vi "DuraFET_pH_CalibCalc.vi"(1 "Eint: (mean voltage)":dbl=0.1318204577803552, 2 "Directemp (C)":dbl, 3 "Eext (REF or Vg)":dbl=1.0) -> (0 "pHint_tot":dbl=9.677584089217062)   [LabVIEW 2018]
panel:
  out "pHext_tot":dbl=nan
  in  "Salinity":dbl
  out "E0ext25":dbl=-inf format="%#_3g"
  out "E0int25":dbl=-0.4202114127602252 format="%#_3g"
  in  "calsal":dbl
  in  "calT":dbl=22.327
  in  "calpH":dbl=9.3
  in  "calEint":dbl=0.127974
  in  "calEext (const)":dbl=1.0
  # "pH Calibration (returns calib. coeff's)"
  # "pH Calculation (returns pHint & pHext)"
  # "INPUTS"
  # "INPUTS"
  # "OUTPUTS"
  # "OUTPUTS"
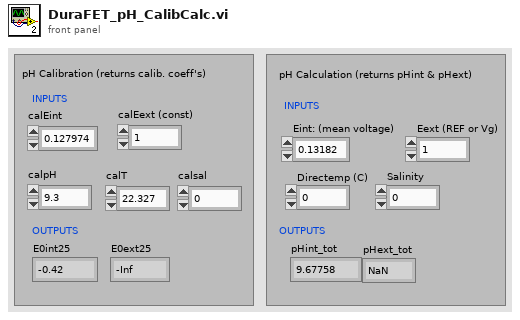
[diagram p1: front panel]
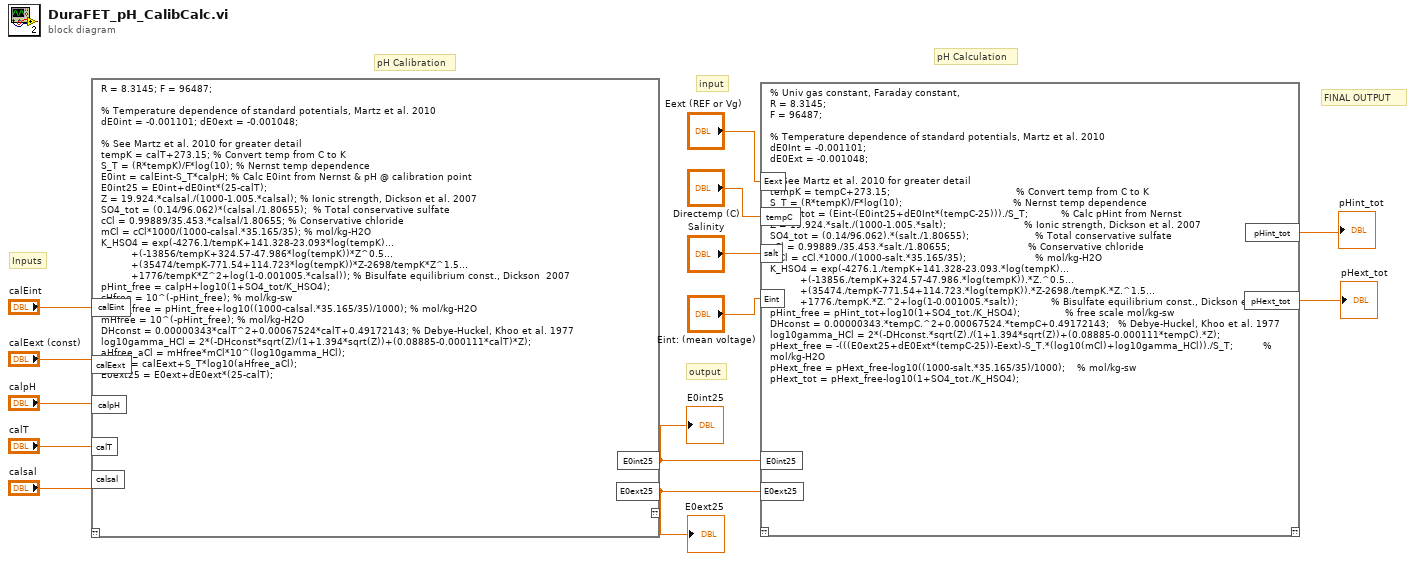
[diagram p0: block diagram]
diagram:
  # "Inputs"
  # "output"
  # "FINAL OUTPUT"
  # "input"
  # "pH Calculation"
  # "pH Calibration"
  n1 = script code="R = 8.3145; F = 96487; \n\n% Temperature dependence of standard potentials, Martz et al. 2010\ndE0int = -0.001101; dE0ext = -0.001048;\n\n% See Martz et al. 2010 for greater detail\ntempK = calT+273.15; % Convert temp from C to K\nS_T = (R*tempK)/F*log(10); % Nernst temp dependence\nE0int = calEint-S_T*calpH; % Calc E0int from Nernst & pH @ calibration point\nE0int25 = E0int+dE0int*(25-calT);\nZ = 19.924.*calsal./(1000-1.005.*calsal); % Ionic strength, Dickson et al. 2007\nSO4_tot = (0.14/96.062)*(calsal./1.80655);  % Total conservative sulfate\ncCl = 0.99889/35.453.*calsal/1.80655; % Conservative chloride\nmCl = cCl*1000/(1000-calsal.*35.165/35); % mol/kg-H2O\nK_HSO4 = exp(-4276.1/tempK+141.328-23.093*log(tempK)...\n          +(-13856/tempK+324.57-47.986*log(tempK))*Z^0.5...\n          +(35474/tempK-771.54+114.723*log(tempK))*Z-2698/tempK*Z^1.5...\n          +1776/tempK*Z^2+log(1-0.001005.*calsal)); % Bisulfate equilibrium const., Dickson  2007\npHint_free = calpH+log10(1+SO4_tot/K_HSO4);\ncHfree = 10^(-pHint_free); % mol/kg-sw\npHint_free = pHint_free+log10((1000-calsal.*35.165/35)/1000); % mol/kg-H2O\nmHfree = 10^(-pHint_free); % mol/kg-H2O\nDHconst = 0.00000343*calT^2+0.00067524*calT+0.49172143; % Debye-Huckel, Khoo et al. 1977\nlog10gamma_HCl = 2*(-DHconst*sqrt(Z)/(1+1.394*sqrt(Z))+(0.08885-0.000111*calT)*Z);\naHfree_aCl = mHfree*mCl*10^(log10gamma_HCl); \nE0ext = calEext+S_T*log10(aHfree_aCl);\nE0ext25 = E0ext+dE0ext*(25-calT);"("calEint"="calEint", "calEext"="calEext (const)", "calpH"="calpH", "calT"="calT", "calsal"="calsal") -> ("E0int25"=w3:cdb, "E0ext25"=w4:cdb)  [unwired: 1 in, 1 out]
  "E0int25" <- w3
  "E0ext25" <- w4
  n2 = script code="% Univ gas constant, Faraday constant, \nR = 8.3145;\nF = 96487; \n\n% Temperature dependence of standard potentials, Martz et al. 2010\ndE0Int = -0.001101; \ndE0Ext = -0.001048;\n\n% See Martz et al. 2010 for greater detail\ntempK = tempC+273.15;                                          % Convert temp from C to K\nS_T = (R*tempK)/F*log(10);                                     % Nernst temp dependence\npHint_tot = (Eint-(E0int25+dE0Int*(tempC-25)))./S_T;           % Calc pHint from Nernst\nZ = 19.924.*salt./(1000-1.005.*salt);                          % Ionic strength, Dickson et al. 2007\nSO4_tot = (0.14/96.062).*(salt./1.80655);                      % Total conservative sulfate\ncCl = 0.99889./35.453.*salt./1.80655;                          % Conservative chloride\nmCl = cCl.*1000./(1000-salt.*35.165/35);                       % mol/kg-H2O\nK_HSO4 = exp(-4276.1./tempK+141.328-23.093.*log(tempK)...\n          +(-13856./tempK+324.57-47.986.*log(tempK)).*Z.^0.5...\n          +(35474./tempK-771.54+114.723.*log(tempK)).*Z-2698./tempK.*Z.^1.5...\n          +1776./tempK.*Z.^2+log(1-0.001005.*salt));           % Bisulfate equilibrium const., Dickson et al. 2007\npHint_free = pHint_tot+log10(1+SO4_tot./K_HSO4);               % free scale mol/kg-sw\nDHconst = 0.00000343.*tempC.^2+0.00067524.*tempC+0.49172143;   % Debye-Huckel, Khoo et al. 1977\nlog10gamma_HCl = 2*(-DHconst.*sqrt(Z)./(1+1.394*sqrt(Z))+(0.08885-0.000111*tempC).*Z);\npHext_free = -(((E0ext25+dE0Ext*(tempC-25))-Eext)-S_T.*(log10(mCl)+log10gamma_HCl))./S_T;          % mol/kg-H2O\npHext_free = pHext_free-log10((1000-salt.*35.165/35)/1000);    % mol/kg-sw\npHext_tot = pHext_free-log10(1+SO4_tot./K_HSO4);"("Eext"="Eext (REF or Vg)", "tempC"="Directemp (C)", "salt"="Salinity", "Eint"="Eint: (mean voltage)", "E0int25"=w3, "E0ext25"=w4) -> ("pHint_tot"=→"pHint_tot":dbl, "pHext_tot"=→"pHext_tot":dbl)  [unwired: 1 in, 1 out]
